vi "Read NET_HttpRequestHeaders.vi"(8 "error in (no error)":errorcluster, 11 "HttpHeaders_Request in":refnum<class "HttpHeaders_Request.lvclass">) -> (0 "error out":errorcluster, 2 "NET_HttpRequestHeaders":refnum<k24>, 3 "HttpHeaders_Request out":refnum<class "HttpHeaders_Request.lvclass">)   [LabVIEW 2018, in "HttpClient_NET.lvlib" / "HttpHeaders_Request.lvclass"]
doc: "<b> </b> <b> </b>\nHttpClient_NET\nJustin Young - Viviota\nCopyright (c) 2021\nLicense: BSD"
uses:
  HttpHeaders_Request.lvclass
  C:/Viviota/Projects/R&D/LabVIEW_HTTP_REST_NET/HTTPHeaders_NET/HttpHeaders_NET.lvclass
  System.Net.Http
  HTTPHeaders_NET/HttpHeaders_NET.lvclass/HttpHeaders_NET.ctl
  HTTPHeaders_NET/HttpHeaders_NET.lvclass
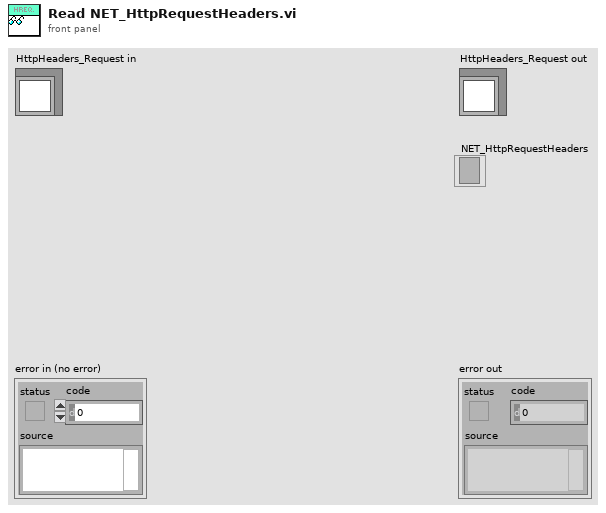
[diagram p1: front panel]
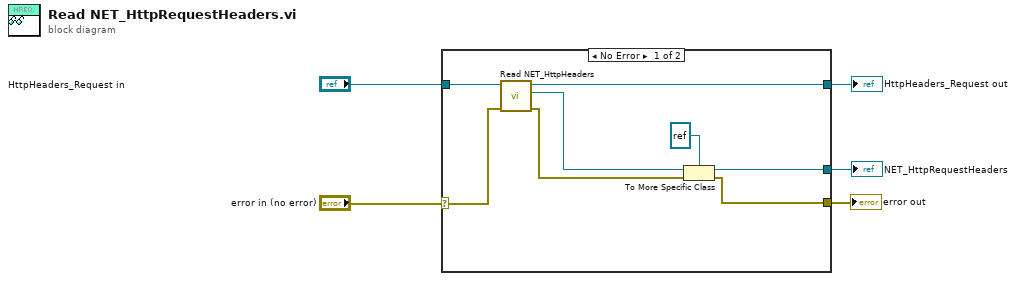
[diagram p0: block diagram]
diagram:
  n1 = case shown="No Error" "error in (no error)" {
    selector: "error in (no error)" -> [w9 w14]
    tunnel: [w6 w14] -> w4
    tunnel: [w10 w15] -> w2
    tunnel: "HttpHeaders_Request in" -> [w11 w15]
    tunnel: [w13 _] -> w1
    frame No Error {
      n2 = call "Read NET_HttpHeaders.vi"("error in (no error)"=w9, "HTTPHeaders_NET in"=w11) -> ("error out"=w7:errorcluster, "NET_HttpHeaders"=w8:refnum<k24>, "HTTPHeaders_NET out"=w10:refnum<class "HttpHeaders_Request.lvclass">)  [unwired: 7 in]
      n3 = To More Specific Class(target class=refnum<k24> refnum ("NET_HttpRequestHeaders"), reference=w8, error in=w7) -> (specific class reference=w13:refnum<k24>, error out=w6:errorcluster)
    }
    frame Error {
    }
  }
  "error out" <- w4
  "HttpHeaders_Request out" <- w2
  "NET_HttpRequestHeaders" <- w1
